vi "DegreesToRadiansSubVI.vi"() -> ()   [LabVIEW 2018]
panel:
  out "Radians":dbl
  in  "Degrees":dbl
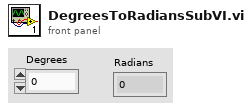
[diagram p1: front panel]
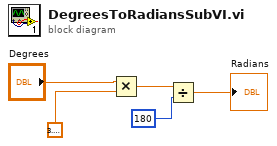
[diagram p0: block diagram]
diagram:
  n1 = Multiply(x="Degrees", y=3.141592653589793) -> (x*y=w3:dbl)
  n2 = Divide(x=w3, y=180) -> (x/y=→"Radians":dbl)
